vi "closeInterface.vi"(6 "error in (no error)":errorcluster, 8 "interface object in":refnum<k20>, 9 "OrionBMS.lvclass":refnum<class "OrionBMSClass.lvclass">) -> (0 "error out":errorcluster, 3 "OrionBMS.lvclass 2":refnum<class "OrionBMSClass.lvclass">)   [LabVIEW 2018, in "OrionBMSClass.lvclass"]
uses:
  OrionBMSClass.lvclass
  <vilib>/CANopenLib/CANOPEN.llb/CANopen Interface Close.vi
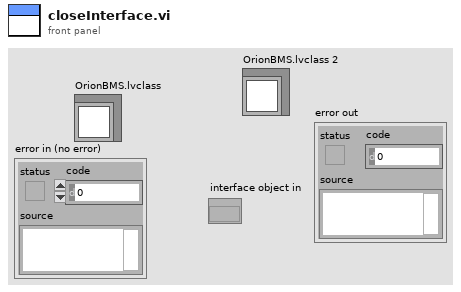
[diagram p1: front panel]
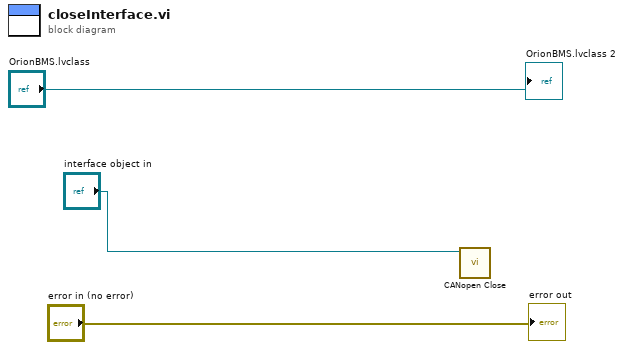
[diagram p0: block diagram]
diagram:
  n1 = call-poly <vilib>:"CANopen Close.vi"("interface object in"="interface object in") -> ()  [unwired: 10 in, 1 out]
  "error out" <- "error in (no error)"
  "OrionBMS.lvclass 2" <- "OrionBMS.lvclass"
